vi "IsFull.vi"(11 "TypedCircularBuffer in":refnum<class "TypedCircularBuffer.lvclass">) -> (2 "Full?":bool, 3 "TypedCircularBuffer out":refnum<class "TypedCircularBuffer.lvclass">)   [LabVIEW 2024, in "TypedCircularBuffer.lvclass"]
uses:
  TypedCircularBuffer.lvclass
  TypedCircularBuffer.lvclass/TypedCircularBuffer.ctl
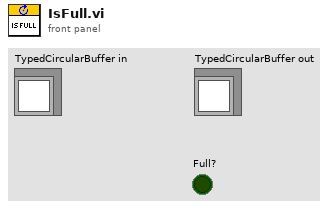
[diagram p1: front panel]
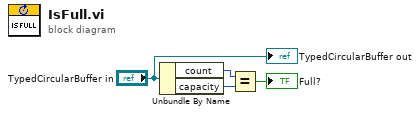
[diagram p0: block diagram]
diagram:
  n1 = Unbundle By Name("TypedCircularBuffer in") -> ("count"=w3:u32, "capacity"=w2:u32)
  n2 = Equal?(x=w3, y=w2) -> (x = y?=→"Full?":bool)
  "TypedCircularBuffer out" <- "TypedCircularBuffer in"
